vi "Get.Flatten.TypeAndData.vi"(4 "PNG U8 Data":u8[](array[numeric])) -> (0 "Payload u8 Data[]":u8[](array[numeric]), 1 "Flat Type":T1=enum."PIX_EXT_FILE", 2 "PNG u8 Data[]":u8[](array[numeric]))   [LabVIEW 2020, in "PixPack.lvlib"]
uses:
  PixPack.lvlib
  Encode.Format.ctl
  32b2b032-07ab-4aaa-9a63-a662edda6e86.vi
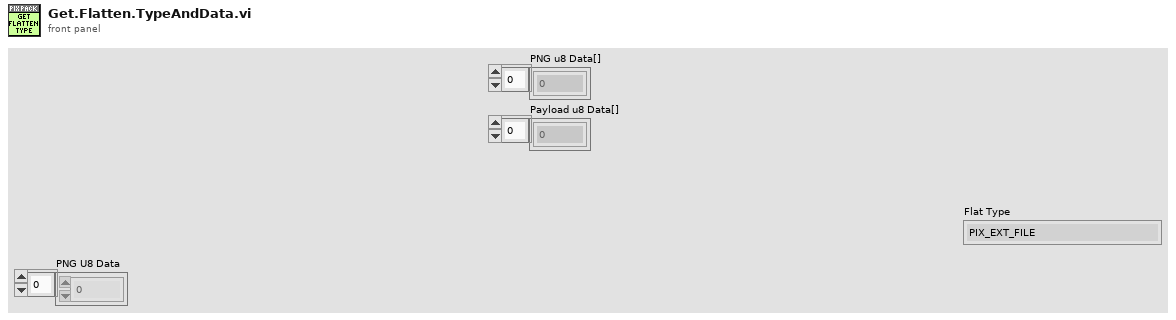
[diagram p1: front panel]
types:
  T1 = typedef "PixPack.lvlib/Encode.Format.ctl" = enum16{"PIX_NOR_FLAT", "PIX_XFLAT", "PIX_EXT_FILE", "PIX_NOT_ENCODED"}
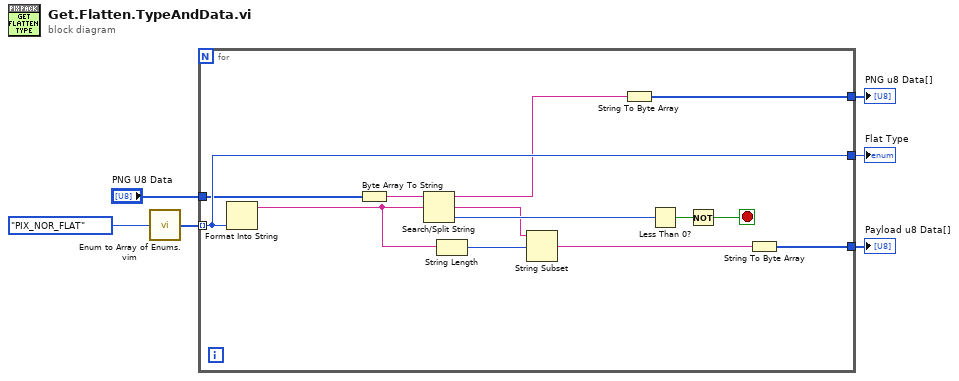
[diagram p0: block diagram]
diagram:
  n1 = call "Enum to Array of Enums.vim"("enum"=Encode.Format."PIX_NOR_FLAT" ("Encode Format")) -> ("array of enums"=w5:T1[])
  n2 = for {
    tunnel: w5 -> [w16] mode=indexing
    tunnel: [w16] -> w3
    tunnel: "PNG U8 Data" -> [w13]
    tunnel: [w7] -> w2
    tunnel: [w9] -> w1
    stop <- w17 stop-if-true
    n3 = Format Into String(w16) -> (resulting string=w11:string)  [unwired: 3 in, 1 out]
    n4 = Byte Array To String(unsigned byte array=w13) -> (string=w12:string)
    n5 = Search/Split String(string=w12, search string/char (-)=w11) -> (substring before match=w8:string, match + rest of string=w14:string, offset of match=w19:i32)  [unwired: 1 in]
    n6 = String Length(string=w11) -> (length=w15:i32)
    n7 = String Subset(string=w14, offset (0)=w15) -> (substring=w10:string)  [unwired: 1 in]
    n8 = String To Byte Array(string=w8) -> (unsigned byte array=w7:u8[])
    n9 = Less Than 0?(x=w19) -> (x < 0?=w18:bool)
    n10 = Not(x=w18) -> (.not. x?=w17:bool)
    n11 = String To Byte Array(string=w10) -> (unsigned byte array=w9:u8[])
  }
  "Flat Type" <- w3
  "PNG u8 Data[]" <- w2
  "Payload u8 Data[]" <- w1
